vi "decimate-points_single_axis.vi"(7 "type":T1, 8 "error in (no error)":errorcluster, 9 "height_width":u32, 10 "y_axis in":dbl[](array[numeric]), 11 "x_axis in":dbl[](array[numeric])) -> (0 "error out":errorcluster, 2 "y_axis out":dbl[](array[numeric]), 3 "x_axis out":dbl[](array[numeric]))   [LabVIEW 2015, in "lv-graph.lvlib"]
doc: "This VI will decimate a given dataset, following the rule that you can display, at most two points per pixel per plot. If the number of points exceeds the number of pixels (wired from height_width). For decimation, it'll group equal sets of points (except the last set) for data representation. As configured, the way the points are represented can be configured as follows: (1) average: this will get the mean of the points per group (2) min_max will average the min/max values for the group (3) max: will return the max value, (4) min: will return the min value, (5) first will return the first value and (6) last will return the last value."
uses:
  lv-graph.lvlib
  _controls/decimation_type.ctl
  <vilib>/Analysis/baseanly.llb/Mean (DBL).vi
  <vilib>/Analysis/NI_AALBase.lvlib
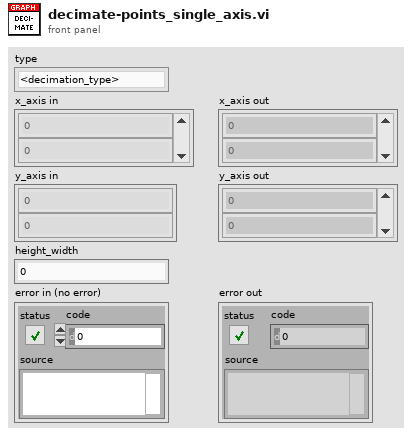
[diagram p1: front panel]
types:
  T1 = typedef "lv-graph.lvlib/decimation_type.ctl" = enum16{"<decimation_type>", "average", "min_max", "max", "min", "first", "last"}
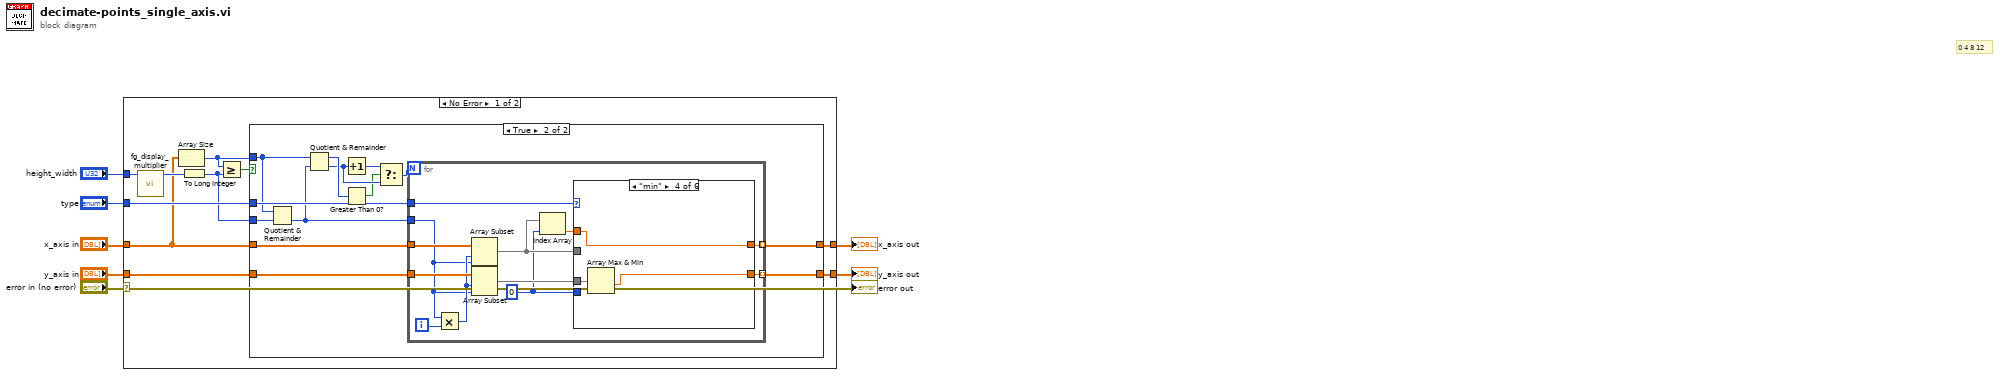
[diagram p0: block diagram]
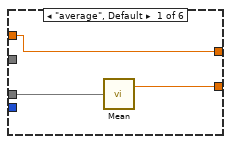
[diagram p3: hidden frame]
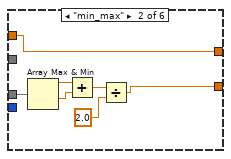
[diagram p4: hidden frame]
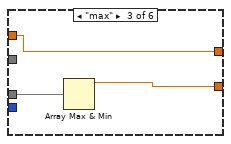
[diagram p5: hidden frame]
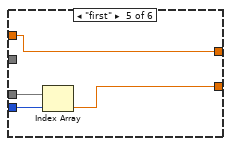
[diagram p6: hidden frame]
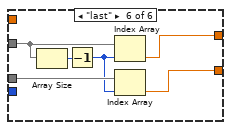
[diagram p7: hidden frame]
diagram:
  # "0 4 8 12"
  n1 = case shown="No Error" "error in (no error)" {
    tunnel: "height_width" -> [w17 _]
    tunnel: "x_axis in" -> [w8 _]
    tunnel: "y_axis in" -> [w16 _]
    tunnel: "type" -> [w15 _]
    tunnel: [w14 _] -> w3
    tunnel: [w13 _] -> w2
    frame No Error {
      n2 = call "fg_display_multiplier.vi"("width_height in"=w17) -> ("width_height out"=w10:u32)  [unwired: 9 in, 1 out]
      n3 = Array Size(array=w8) -> (size(s)=w12:i32)
      n4 = To Long Integer(number=w10) -> (32bit integer=w9:i32)
      n5 = Greater Or Equal?(x=w12, y=w9) -> (x >= y?=w11:bool)
      n6 = case shown="True" w11 {
        tunnel: w8 -> [w19 w28]
        tunnel: w16 -> [w18 w27]
        tunnel: w15 -> [_ w26]
        tunnel: w12 -> [_ w21]
        tunnel: w9 -> [_ w25]
        tunnel: [w19 w24] -> w14
        tunnel: [w18 w20] -> w13
        frame False {
        }
        frame True {
          n7 = Quotient & Remainder(x=w21, y=w25) -> (floor(x/y)=w22:i32)  [unwired: 1 out]
          n8 = Quotient & Remainder(x=w21, y=w22) -> (x-y*floor(x/y)=w32:i32, floor(x/y)=w31:i32)
          n9 = Increment(x=w31) -> (x+1=w29:i32)
          n10 = Greater Than 0?(x=w32) -> (x > 0?=w23:bool)
          n11 = Select(t=w29, s=w23, f=w31) -> (s? t:f=w30:i32)
          n12 = for {
            N: w30 -> [_]
            tunnel: w22 -> [w36]
            tunnel: w28 -> [w42]
            tunnel: w27 -> [w44]
            tunnel: w26 -> [w39]
            tunnel: [w41] -> w20 mode=indexing
            tunnel: [w40] -> w24 mode=indexing
            i -> [w43]
            w33 = 0 ("index")
            n13 = Multiply(x=w36, y=w43) -> (x*y=w37:i32)
            n14 = Array Subset(array=w42, index=w37, length=w36) -> (w35:dbl[])
            n15 = Array Subset(array=w44, index=w37, length=w36) -> (w38:dbl[])
            n16 = Index Array(array=w35, index=w33) -> (element=w34:dbl)
            n17 = case shown="\"min\"" w39 {
              tunnel: w35 -> [_ _ _ _ _ w68]
              tunnel: w38 -> [w47 w54 w57 w60 w64 w66]
              tunnel: [w46 w53 w56 w59 w63 w69] -> w41
              tunnel: [w45 w48 w55 w58 w61 w70] -> w40
              tunnel: w34 -> [w45 w48 w55 w58 w61 _]
              tunnel: w33 -> [_ _ _ _ w62 _]
              frame "average", Default {
                n18 = call-poly <vilib>:"Mean.vi"("X"=w47) -> ("mean"=w46:dbl)  [unwired: 1 out]
              }
              frame "min_max" {
                n19 = Array Max & Min(array=w54) -> (max value=w52:dbl, min value=w51:dbl)  [unwired: 2 out]
                n20 = Add(x=w52, y=w51) -> (x+y=w50:dbl)
                n21 = Divide(x=w50, y=2.0) -> (x/y=w53:dbl)
              }
              frame "max" {
                n22 = Array Max & Min(array=w57) -> (max value=w56:dbl)  [unwired: 3 out]
              }
              frame "min" {
                n23 = Array Max & Min(array=w60) -> (min value=w59:dbl)  [unwired: 3 out]
              }
              frame "first" {
                n24 = Index Array(array=w64, index=w62) -> (element=w63:dbl)
              }
              frame "last" {
                n25 = Array Size(array=w68) -> (size(s)=w67:i32)
                n26 = Decrement(x=w67) -> (x-1=w65:i32)
                n27 = Index Array(array=w68, index=w65) -> (element=w70:dbl)
                n28 = Index Array(array=w66, index=w65) -> (element=w69:dbl)
              }
            }
          }
        }
      }
    }
    frame Error {
    }
  }
  "x_axis out" <- w3
  "y_axis out" <- w2
  "error out" <- "error in (no error)"
